vi "LoadNew2DGraph_LS1.vi"(5 "MainGraphQ":refnum<queue>, 7 "GraphEvent":refnum<user-event>, 8 "ErrorIn(No Error)":errorcluster caption="entrée d'erreur (pas d'erreur)", 9 "GraphIndex":i32) -> (0 "sortie d'erreur":errorcluster, 1 "Graph":refnum<vi>, 2 "2DGraphQRef":refnum<queue>)   [LabVIEW 2019]
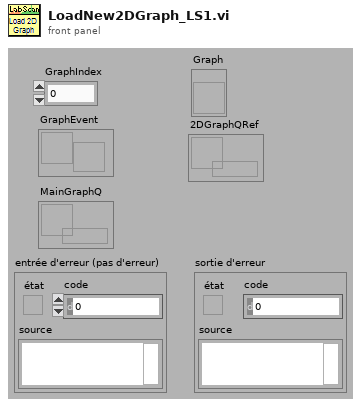
[diagram p1: front panel]
types:
  T1 = enum32{"Invalid", "Standard", "Closed", "Hidden", "Minimized", "Maximized"}
  T2 = enum16{"Répertoire du VI actuel", "Répertoire du parent 1", "Répertoire du parent 2", "Répertoire du parent 3"}
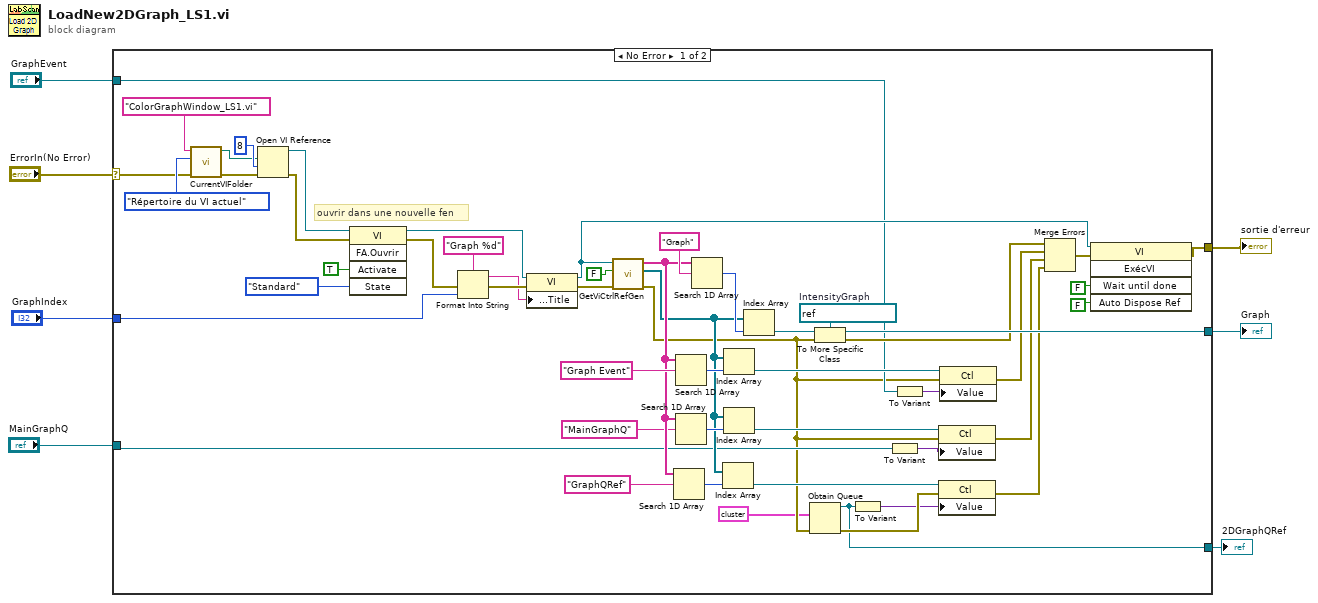
[diagram p0: block diagram]
diagram:
  n1 = case shown="No Error" "ErrorIn(No Error)" {
    selector: "ErrorIn(No Error)" -> [w57 w60]
    tunnel: [w28 w60] -> w6
    tunnel: [w50 _] -> w5
    tunnel: "GraphIndex" -> [w44 _]
    tunnel: "GraphEvent" -> [w24 _]
    tunnel: "MainGraphQ" -> [w17 _]
    tunnel: [w13 _] -> w1
    frame No Error {
      w49 = refnum<vi> refnum  # IntensityGraph
      # "ouvrir dans une nouvelle fen"
      n2 = call <userlib>:"CurrentVIFolder.vi"("error in (no error)"=w57, "Source"=T2."Répertoire du VI actuel", "NomFichier"="ColorGraphWindow_LS1.vi") -> ("error out"=w59:errorcluster, "Chemin"=w31:path)  [unwired: 6 in, 1 out]
      n3 = Open VI Reference(vi path=w31, options=8, error in (no error)=w59) -> (vi reference=w48:refnum<vi>, error out=w55:errorcluster)  [unwired: 3 in]
      n4 = invoke class="VI" method="FA.Ouvrir"(reference=w48, error in=w55, "Activate"=TRUE ("Activer ?"), "State"=T1."Standard" ("État")) -> (reference out=w30:refnum<vi>, error out=w25:errorcluster)  [unwired: 1 in, 3 out]
      n5 = Format Into String(format string="Graph %d" ("chaîne de format"), error in=w25, w44) -> (resulting string=w26:string, error out=w42:errorcluster)  [unwired: 1 in]
      n6 = property class="VI"(reference=w30, error in=w42, "Front Panel.Title"=w26) -> (reference out=w27:refnum<vi>, error out=w45:errorcluster)
      n7 = call <userlib>:"GetViCtrlRefGen.vi"("ErrorIn(No Error)"=w45, "InclTabCTrl"=FALSE, "VIRef"=w27) -> ("sortie d'erreur"=w9:errorcluster, "ControlsRefs"=w21:refnum<vi>[], "ControlsNames"=w22:string[])  [unwired: 6 in]
      n8 = Search 1D Array(1D array=w22, element="GraphQRef" ("élément")) -> (index of element=w35:i32)  [unwired: 1 in]
      n9 = Search 1D Array(1D array=w22, element="Graph Event" ("élément")) -> (index of element=w39:i32)  [unwired: 1 in]
      n10 = Search 1D Array(1D array=w22, element="MainGraphQ" ("élément")) -> (index of element=w23:i32)  [unwired: 1 in]
      n11 = Search 1D Array(1D array=w22, element="Graph" ("élément")) -> (index of element=w52:i32)  [unwired: 1 in]
      n12 = Index Array(array=w21, index=w35) -> (element=w33:refnum<vi>)
      n13 = Index Array(array=w21, index=w39) -> (element=w38:refnum<vi>)
      n14 = Index Array(array=w21, index=w23) -> (element=w19:refnum<vi>)
      n15 = Index Array(array=w21, index=w52) -> (element=w51:refnum<vi>)
      n16 = Obtain Queue(element data type=cluster{"Message":string, "Data":variant, i32} {"Message"="", "Data"=variant, 0} ("élément"), error in (no error)=w9) -> (queue out=w13:refnum<queue>, error out=w32:errorcluster)  [unwired: 3 in, 1 out]
      n17 = To More Specific Class(target class=w49, reference=w51, error in=w9) -> (specific class reference=w50:refnum<vi>, error out=w41:errorcluster)
      n18 = To Variant(anything=w13) -> (Variant=w14:variant)
      n19 = To Variant(anything=w17) -> (Variant=w20:variant)
      n20 = To Variant(anything=w24) -> (Variant=w37:variant)
      n21 = property class="Ctl"(reference=w19, error in=w9, "Value"=w20) -> (error out=w16:errorcluster)  [unwired: 1 out]
      n22 = property class="Ctl"(reference=w33, error in=w32, "Value"=w14) -> (error out=w15:errorcluster)  [unwired: 1 out]
      n23 = property class="Ctl"(reference=w38, error in=w9, "Value"=w37) -> (error out=w36:errorcluster)  [unwired: 1 out]
      n24 = Merge Errors(w41, w36, w16, w15) -> (w29:errorcluster)
      n25 = invoke class="VI" method="ExécVI"(reference=w27, error in=w29, "Wait until done"=FALSE ("Attendre la fin"), "Auto Dispose Ref"=FALSE ("Supprimer la référence automatiquement")) -> (error out=w28:errorcluster)  [unwired: 1 in, 4 out]
    }
    frame Error {
    }
  }
  "sortie d'erreur" <- w6
  "Graph" <- w5
  "2DGraphQRef" <- w1
